vi "Serialize.vi"(8 "error in (no error)":errorcluster, 11 "RandomNumberGenerator Controller in":refnum<class "RandomNumberGenerator Controller.lvclass">) -> (0 "error out":errorcluster, 2 "Serialized PE Specification":string, 3 "RandomNumberGenerator Controller out":refnum<class "RandomNumberGenerator Controller.lvclass">)   [LabVIEW 2020, in "RandomNumberGenerator.lvlib" / "RandomNumberGenerator Controller.lvclass"]
doc: "<b>Serialize</b>\nProvides the seralized configuration data stored in the plugin controller's class data."
uses:
  RandomNumberGenerator Controller.lvclass
  RandomNumberGenerator Controller.lvclass/RandomNumberGenerator Controller.ctl
  PE/Get Configuration Version.vi
  <vilib>/ADAS Record/Utilities/Config/Data Converter/Data Container and Version to JSON.vi
  PE/RandomNumberGenerator.lvclass
panel:
  # "#via_ignore"
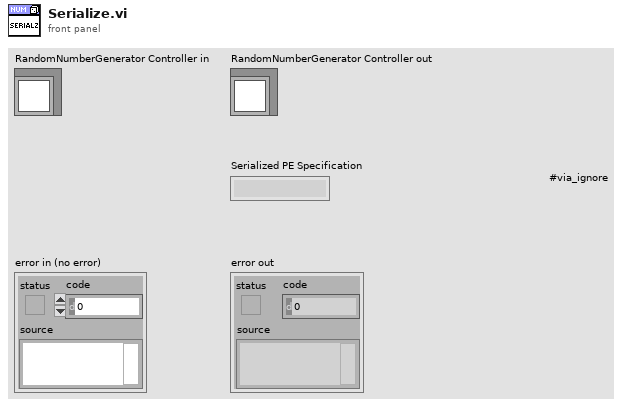
[diagram p1: front panel]
types:
  T1 = typedef "RandomNumberGenerator.lvlib/RandomNumberGenerator.lvclass/Configuration.ctl" = cluster{"Parameter1":string}
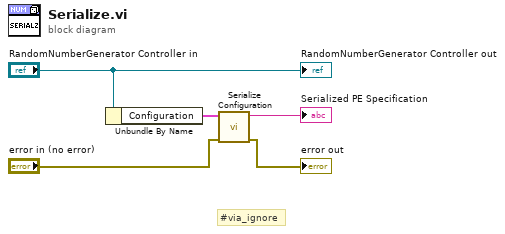
[diagram p0: block diagram]
diagram:
  # "#via_ignore"
  n1 = Unbundle By Name("RandomNumberGenerator Controller in") -> ("Configuration"=w4:T1)
  n2 = call "Serialize Configuration.vi"("error in (no error)"="error in (no error)", "Configuration"=w4) -> ("error out"=→"error out":errorcluster, "Serialized Configuration"=→"Serialized PE Specification":string)  [unwired: 8 in]
  "RandomNumberGenerator Controller out" <- "RandomNumberGenerator Controller in"
